vi "GUID to U8 GUID.vi"(8 "error in (no error)":errorcluster, 11 "GUID In":string) -> (0 "error out":errorcluster, 3 "U8 GUID":u8[](array[numeric]) format="%.0x")   [LabVIEW 2021, in "DataTypes_CIF_U.lvlib"]
doc: "A GUID is a string representation of the hex values of 16 bytes. This converts a string GUID to the 16 bytes."
uses:
  DataTypes_CIF_U.lvlib
  Typedef/Errors.ctl
  Errors/Append Error Location.vi
  <vilib>/regexp/Match Regular Expression.xnode
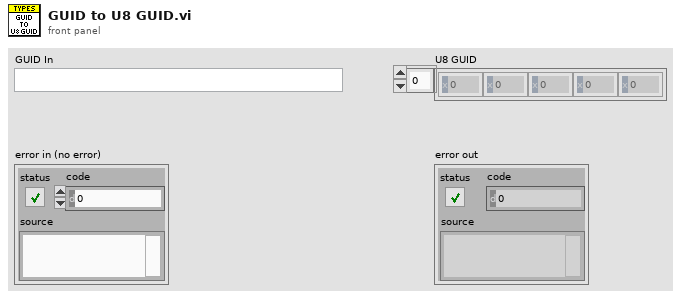
[diagram p1: front panel]
types:
  T1 = typedef "DataTypes_CIF_U.lvlib/Errors.ctl" = enum16{"Too few bytes", "Unsupported Type", "Invalid GUID"}
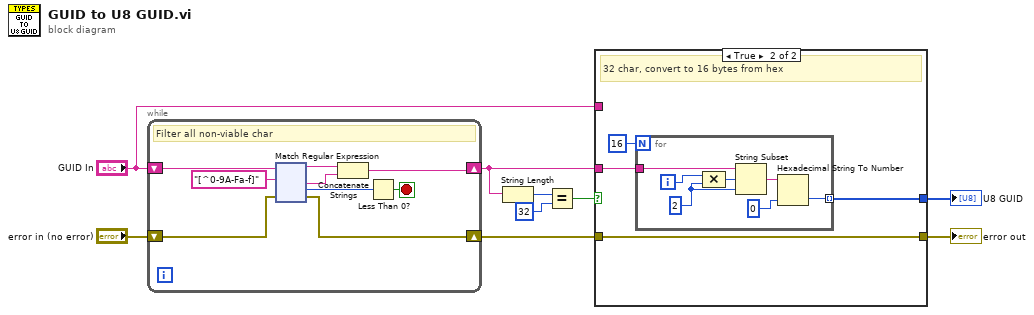
[diagram p0: block diagram]
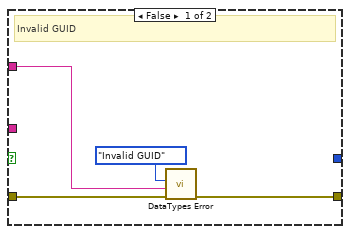
[diagram p2: hidden frame]
diagram:
  n1 = while {
    shift-right: [w12] -> w6
    shift-left: "GUID In" -> [w17]
    shift-right: [w10] -> w4
    shift-left: "error in (no error)" -> [w11]
    stop <- w13 stop-if-true
    # "Filter all non-viable char"
    n2 = xnode "Match Regular Expression"("input string"=w17, "regular expression"="[^0-9A-Fa-f]", "error in"=w11) -> ("before match"=w16:string, "after match"=w15:string, "offset past match"=w14:i32, "error out"=w10:errorcluster)  [unwired: 3 in, 1 out]
    n3 = Concatenate Strings(w16, w15) -> (w12:string)
    n4 = Less Than 0?(x=w14) -> (x < 0?=w13:bool)
  }
  n5 = String Length(string=w6) -> (length=w9:i32)
  n6 = Equal?(x=w9, y=32) -> (x = y?=w7:bool)
  n7 = case shown="True" w7 {
    tunnel: w6 -> [_ w142]
    tunnel: [_ w141] -> w3
    tunnel: w4 -> [w139 w140]
    tunnel: [w138 w140] -> w2
    tunnel: "GUID In" -> [w137 _]
    frame False {
      # "Invalid GUID"
      n8 = call "DataTypes Error.vi"("error in (no error)"=w139, "String to Append"=w137, "Error"=Errors."Invalid GUID") -> ("error out"=w138:errorcluster)  [unwired: 8 in]
    }
    frame True {
      # "32 char, convert to 16 bytes from hex"
      n9 = for {
        N: 16 -> [_]
        tunnel: w142 -> [w148]
        tunnel: [w149] -> w141 mode=indexing
        i -> [w144]
        w145 = 2 ("x")
        n10 = Compound Arithmetic op=MULTIPLY(w144, w145) -> (w146:i32)
        n11 = String Subset(string=w148, offset (0)=w146, length (rest)=w145) -> (substring=w147:string)
        n12 = Hexadecimal String To Number(string=w147, default (0uL)=u8 0) -> (number=w149:u8)  [unwired: 1 in, 1 out]
      }
    }
  }
  "U8 GUID" <- w3
  "error out" <- w2
